vi "Set Pin Map ID for Sequence.vi"(8 "error in":errorcluster, 10 "pin_map_id":string, 11 "sequence context in":refnum<k7>) -> (0 "error out":errorcluster, 3 "sequence context out":refnum<k7>)   [LabVIEW 2020, in "MeasurementLink Pin Map.lvlib"]
doc: "Sets the pin map ID for a TestStand sequence."
uses:
  MeasurementLink Pin Map.lvlib
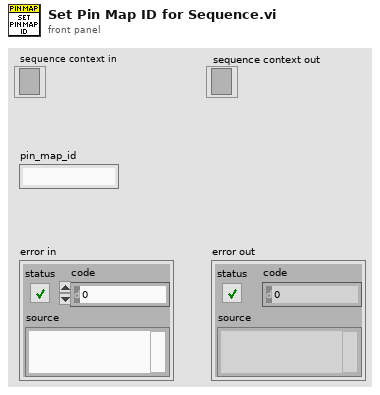
[diagram p1: front panel]
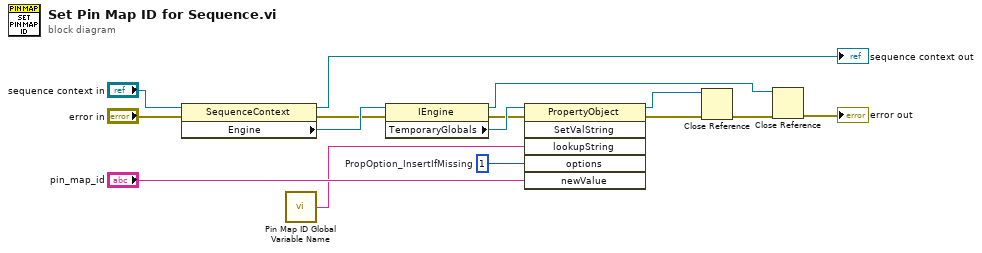
[diagram p0: block diagram]
diagram:
  w3 = 1  # PropOption_InsertIfMissing
  n1 = property class="SequenceContext"(reference="sequence context in", error in="error in") -> (reference out=→"sequence context out":refnum<k7>, error out=w7:errorcluster, "Engine"=w9:refnum<k7>)
  n2 = call "Pin Map ID Global Variable Name.vi"() -> ("global variable name"=w1:string)
  n3 = property class="IEngine"(reference=w9, error in=w7) -> (reference out=w13:refnum<k7>, error out=w5:errorcluster, "TemporaryGlobals"=w10:refnum<k7>)
  n4 = invoke class="PropertyObject" method="SetValString"(reference=w10, error in=w5, "lookupString"=w1, "options"=w3, "newValue"="pin_map_id") -> (reference out=w11:refnum<k7>, error out=w12:errorcluster)  [unwired: 1 in, 4 out]
  n5 = Close Reference(reference=w11, error in (no error)=w12) -> (error out=w14:errorcluster)
  n6 = Close Reference(reference=w13, error in (no error)=w14) -> (error out=→"error out":errorcluster)
